vi "Get Property.vi"(8 "error in (no error)":errorcluster caption="错误输入（无错误）", 9 "Default Value":variant, 10 "Property Name":string, 11 "Item输入":refnum<class "Item.lvclass">) -> (0 "error out":errorcluster caption="错误输出", 1 "Value":variant, 3 "Item输出":refnum<class "Item.lvclass">, 4 "found":bool)   [LabVIEW 2013, in "Hierarchy Framework.lvlib" / "Item.lvclass"]
doc: "Returns the <B>Value</B> of a specific item <B>Property Name</B>. Properties do not inherit within a custom device, so <B>Item Ref in</B> must reference the specific item on which the property is set. \n\nFor instances with a <B>Default Value</B> input, the <B>Value</B> output returns this value if the <B>Property Name</B> is not found for the specified item. Wire data to the <B>Default Value</B> input to determine the polymorphic instance to use or manually select the instance."
uses:
  Item.lvclass
  Item.lvclass/Item.ctl
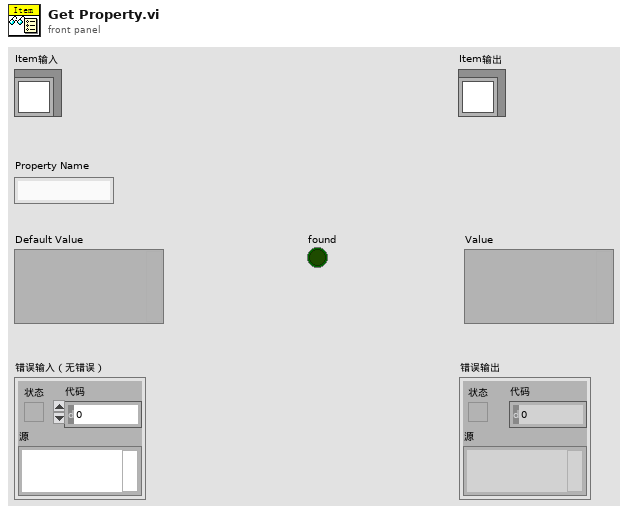
[diagram p1: front panel]
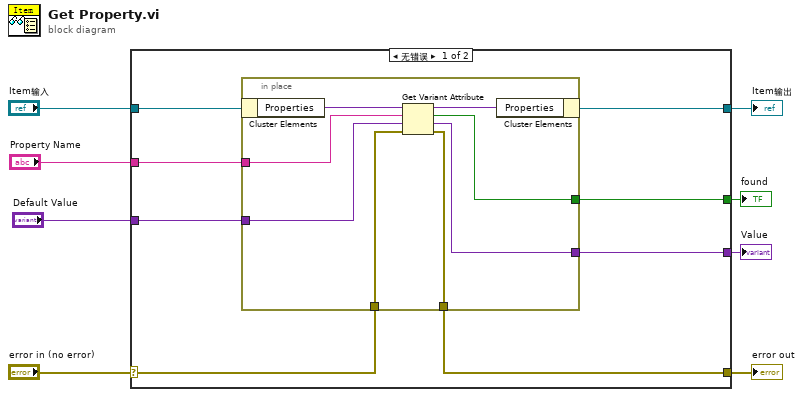
[diagram p0: block diagram]
diagram:
  n1 = case shown="无错误" "error in (no error)" {
    selector: "error in (no error)" -> [w12 w27]
    tunnel: [w11 w27] -> w7
    tunnel: [w15 w26] -> w5
    tunnel: "Item输入" -> [w16 w26]
    tunnel: "Property Name" -> [w14 _]
    tunnel: "Default Value" -> [w13 w25]
    tunnel: [w10 w25] -> w2
    tunnel: [w9 _] -> w1
    frame No Error {
      n2 = in-place {
        in-place-border: [w22] -> w9
        in-place-border: w14 -> [w21]
        in-place-border: w13 -> [w20]
        in-place-border: w12 -> [w19]
        in-place-border: [w18] -> w11
        in-place-border: [w17] -> w10
        n3 = in-place-cluster #1(w16) -> ("Properties"=w24:variant)
        n4 = Get Variant Attribute(Variant=w24, name=w21, default value (empty Variant)=w20, error in=w19) -> (duplicate Variant=w23:variant, found=w22:bool, value=w17:variant, error out=w18:errorcluster)
        n5 = in-place-cluster #1("Properties"=w23) -> (w15:refnum<class "Item.lvclass">)
      }
    }
    frame Error {
    }
  }
  "error out" <- w7
  "Item输出" <- w5
  "Value" <- w2
  "found" <- w1
